vi "ATF-Connect RT.vi"(7 "PUMP IP":string="LOCALHOST", 8 "error in (no error)":errorcluster, 9 "STORAGE IP":string, 10 "Select type":T1, 11 "?":T2) -> (0 "error out":errorcluster, 3 "?":T2)   [LabVIEW 2022 SP3]
uses:
  Controls/main case.ctl
  Controls/SeCrTs-boolean ref.ctl
  Controls/SeCrTs-EPV .ctl
  Controls/Commands to log.ctl
  UI Message handler/Message Queue/All Message Queues.ctl
  UI Message handler/Message Queue/Message Cluster.ctl
  Controls/SeCrTs-Notifier ctl.ctl
  Controls/SeCrTs-NS Data type.ctl
  Controls/ATF-Select device.ctl
  UI Message handler/Message Queue/Message Queue.lvlib
types:
  T1 = typedef "ATF-Select device.ctl" = enum16{"All", "Pump", "Storage"}
  T2 = typedef "main case.ctl" = cluster{"Bol":T3, "EPV":T4, "Covers":cluster{"cover":refnum<vi>, "Login screen cover":refnum<vi>, "cover Motor":refnum<vi>, "PPSU cover":refnum<vi>}, "Log cmd":T5, "STORAGE IP":string, "PUMP IP":string, "Storage con":bool, "Pumb con":bool, "que ref":T6, "not ref":T7, "notification":cluster{"C/NC":bool, "Start/Stop Log":bool[], "Log Name":string, "Config":cluster{"AO config":cluster{"Channel_Name":string, "Channel_Number":string, "Default_Value":dbl, "Units":string}[], "AI config":cluster{"Channel_Name":string, "Channel_Number":string, "Pre_Scale_min":dbl, "Pre_Scale_max":dbl, "Sensor_min":dbl, "Sensor_max":dbl, "Units":string}[], "DI config":cluster{"Channel_Name":string, "Channel_Number":string, "Default_Value":bool, "DI invert?":bool}[], "DO config":cluster{"Channel_Name":string, "Channel_Number":string, "Default_Value":bool, "DO invert?":bool}[], "TC config":cluster{"Channel_Name":string, "Channel_Number":string, "Pre_Scale_min":dbl, "Pre_Scale_max":dbl, "units":i32, " type":i32}[], "ACC config":cluster{"Channel_Name":string, "Channel_Number":string, "Pre_Scale_min":dbl, "Pre_Scale_max":dbl, "Terminal configuration":i32, "Sensitivity":dbl, "Sensitivity units":i32}[], "SG config":cluster{"Channel_Name":string, "Channel_Number":string, "Pre_Scale_min":dbl, "Pre_Scale_max":dbl}[], "Strain Gauge Settings":cluster{"poisson ratio":dbl, "nominal gage resistance":dbl, "gage factor":dbl}, "Bridge Settings":cluster{"voltage excitation value":dbl, "voltage excitation source":i32, "initial bridge voltage":dbl, "lead wire resistance":dbl, "strain configuration":i32}, "Sample Rate":cluster{"AI Sample Rate":dbl[], "AO Sample Rate":dbl[], "DI Sample Rate":dbl[], "TC Sample Rate":dbl[], "DO Sample Rate":dbl[], "SG Sample Rate":dbl[], "ACC Sample Rate":dbl[]}, "Drive":cluster{"Drive_Health":bool, "Drive_Frequency":u32, "Drive_Status":bool, "Drive_RPM":u32, "Drive_Direction":bool, "Acceleration state":bool, "Steady state":bool, "Deceleration state":bool, "Drive_Enable":bool, "Drive set_RPM":dbl}}, "Log min":dbl}, "Exit Drive ATF":refnum<vi>}
  T3 = typedef "SeCrTs-boolean ref.ctl" = cluster{"Connect RT":refnum<vi>, "START DAQ":refnum<vi>, "STOP DAQ":refnum<vi>, "DAQ SETTING":refnum<vi>, "START LOG":refnum<vi>, "STOP LOG":refnum<vi>, "Connect Drive ATF":refnum<vi>, "Update drive ATF":refnum<vi>, "Gate driver ATF":refnum<vi>, "Motor On ATF":refnum<vi>, "ADC reset ATF":refnum<vi>, "Gate driver ATF 2":refnum<vi>, "Motor off ATF":refnum<vi>, "MCU reset ATF":refnum<vi>, "Connect Drive Lox":refnum<vi>, "Update drive lox":refnum<vi>, "Gate driver- LOX":refnum<vi>, "Motor On lox":refnum<vi>, "Adc reset lox":refnum<vi>, "MCU Reset -LOX":refnum<vi>, "Motor Off lox":refnum<vi>, "Connect ppsu":refnum<vi>, "update ppsu":refnum<vi>, "DC on":refnum<vi>, "Alarm ack":refnum<vi>, "DC off":refnum<vi>, "Ms initialize":refnum<vi>, "Exit RT":refnum<vi>, "ABORT":refnum<vi>, "HOLD UPDATE":refnum<vi>, "Log type":refnum<vi>, "PUMP IP":refnum<vi>, "STORAGE IP":refnum<vi>}
  T4 = typedef "SeCrTs-EPV .ctl" = cluster{"F_EPV_131":refnum<vi>, "F_EPV_132":refnum<vi>, "F_EPV_136":refnum<vi>, "F_EPV_21":refnum<vi>, "F_EPV_41":refnum<vi>, "N_EPV_68":refnum<vi>, "N_EPV_ 69":refnum<vi>, "N_EPV_ 33":refnum<vi>, "F_EPV_142":refnum<vi>, "F_EPV_28":refnum<vi>, "N_EPV_203":refnum<vi>, "N_EPV_206":refnum<vi>, "F_EPV_75":refnum<vi>, "C_EPV_2":refnum<vi>, "C_EPV_7":refnum<vi>, "C_EPV_8":refnum<vi>, "C_EPV_123":refnum<vi>, "C_EPV_124":refnum<vi>, "C_EPV_127":refnum<vi>, "N_EPV_62a":refnum<vi>, "N_EPV_62b":refnum<vi>, "N_EPV_61":refnum<vi>, "G_EPV_51":refnum<vi>, "N_EPV_141":refnum<vi>, "C_EPV_803":refnum<vi>, "C_EPV_18":refnum<vi>, "C_EPV_1352":refnum<vi>, "N_EPV_202":refnum<vi>, "C_EPV_16":refnum<vi>}
  T5 = typedef "Commands to log.ctl" = cluster{"C/NC":bool, "Start/Stop Log":bool[], "Log Name":string, "Config":cluster{"AO config":cluster{"Channel_Name":string, "Channel_Number":string, "Default_Value":dbl, "Units":string}[], "AI config":cluster{"Channel_Name":string, "Channel_Number":string, "Pre_Scale_min":dbl, "Pre_Scale_max":dbl, "Sensor_min":dbl, "Sensor_max":dbl, "Units":string}[], "DI config":cluster{"Channel_Name":string, "Channel_Number":string, "Default_Value":bool, "DI invert?":bool}[], "DO config":cluster{"Channel_Name":string, "Channel_Number":string, "Default_Value":bool, "DO invert?":bool}[], "TC config":cluster{"Channel_Name":string, "Channel_Number":string, "Pre_Scale_min":dbl, "Pre_Scale_max":dbl, "units":i32, " type":i32}[], "ACC config":cluster{"Channel_Name":string, "Channel_Number":string, "Pre_Scale_min":dbl, "Pre_Scale_max":dbl, "Terminal configuration":i32, "Sensitivity":dbl, "Sensitivity units":i32}[], "SG config":cluster{"Channel_Name":string, "Channel_Number":string, "Pre_Scale_min":dbl, "Pre_Scale_max":dbl}[], "Strain Gauge Settings":cluster{"poisson ratio":dbl, "nominal gage resistance":dbl, "gage factor":dbl}, "Bridge Settings":cluster{"voltage excitation value":dbl, "voltage excitation source":i32, "initial bridge voltage":dbl, "lead wire resistance":dbl, "strain configuration":i32}, "Sample Rate":cluster{"AI Sample Rate":dbl[], "AO Sample Rate":dbl[], "DI Sample Rate":dbl[], "TC Sample Rate":dbl[], "DO Sample Rate":dbl[], "SG Sample Rate":dbl[], "ACC Sample Rate":dbl[]}}, "Log min":dbl, "Drive":cluster{"Drive_Health":bool, "Drive_Frequency":u32, "Drive_Status":bool, "Drive_RPM":u32, "Drive_Direction":bool, "Acceleration state":bool, "Steady state":bool, "Deceleration state":bool, "Drive_Enable":bool, "Drive set_RPM":dbl}, "HOLD UPDATE":bool}
  T6 = typedef "Message Queue.lvlib/All Message Queues.ctl" = cluster{"UI":refnum<queue>, "ER":refnum<queue>, "Ev":refnum<queue>, "R ER Storage":refnum<queue>, "PPSU":refnum<queue>, "R ER Pumb":refnum<queue>}
  T7 = typedef "SeCrTs-Notifier ctl.ctl" = cluster{"Storage Data":refnum<notifier>, "Pumb Data":refnum<notifier>, "Log cmd":refnum<notifier>}
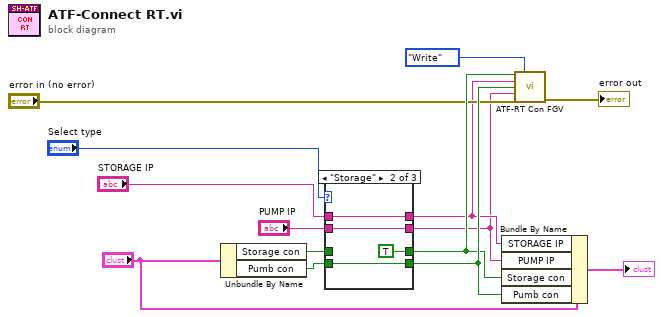
[diagram p0: block diagram]
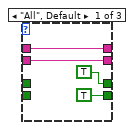
[diagram p2: hidden frame]
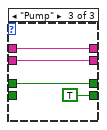
[diagram p3: hidden frame]
diagram:
  n1 = Unbundle By Name("?") -> ("Storage con"=w10:bool, "Pumb con"=w11:bool)
  n2 = case shown="\"Storage\"" "Select type" {
    tunnel: [w16 w21 w26] -> w2
    tunnel: [TRUE ("Storage rt con") TRUE ("Storage rt con") w23] -> w12
    tunnel: "STORAGE IP" -> [w16 w21 w26]
    tunnel: "PUMP IP" -> [w15 w20 w25]
    tunnel: [w15 w20 w25] -> w1
    tunnel: [TRUE ("Pumb rt con") w19 TRUE ("Pumb rt con")] -> w13
    tunnel: w10 -> [_ _ w23]
    tunnel: w11 -> [_ w19 _]
    frame "All", Default {
    }
    frame "Storage" {
    }
    frame "Pump" {
    }
  }
  n3 = Bundle By Name(cluster="?", "STORAGE IP"=w2, "PUMP IP"=w1, "Storage con"=w12, "Pumb con"=w13) -> (→"?":T2)
  n4 = call "ATF-RT Con FGV.vi"("Storage rt con"=w12, "Enum"=enum16{"Read", "Write"}."Write", "Storage IP"=w2, "Pumb rt con"=w13, "Pump IP"=w1, "error in"="error in (no error)") -> ("error out"=→"error out":errorcluster)  [unwired: 5 in, 4 out]
